vi "Reset To Temporary Passwordvi.vi"(0 "User Configuration Manager in":refnum<class "User Configuration Manager.lvclass">, 5 "Username":string, 11 "error in (no error)":errorcluster) -> (4 "User Configuration Manager out":refnum<class "User Configuration Manager.lvclass">, 6 "User Found":bool, 8 "Temporary Password":string, 15 "error out":errorcluster)   [LabVIEW 2020, in "User Configuration Manager.lvlib" / "User Configuration Manager.lvclass"]
doc: "Resets the password of the user specified by user name to a temporary password."
uses:
  <vilib>/gpm_packages/@cs/user-manager/Source/User Configuration Manager/User Configuration Manager.lvclass
  <vilib>/gpm_packages/@cs/user-manager/Source/User Configuration Manager/User Configuration Manager.lvclass/User Configuration Manager.ctl
  1ef86e87-005e-4bc9-afcc-fd6cee3e8d09.vi
  <vilib>/gpm_packages/@cs/user-manager/Source/User Configuration Manager/Accessors/Read Linked List Ref .vi
  <vilib>/gpm_packages/@cs/user-manager/Source/User Configuration Manager/Read Encryption Type.vi
  <vilib>/gpm_packages/@cs/linked-list/Source/Linked List/ILinkedList/ILinked List.lvclass
  <vilib>/gpm_packages/@cs/user-manager/Source/iEncryption/iEncryption.lvclass
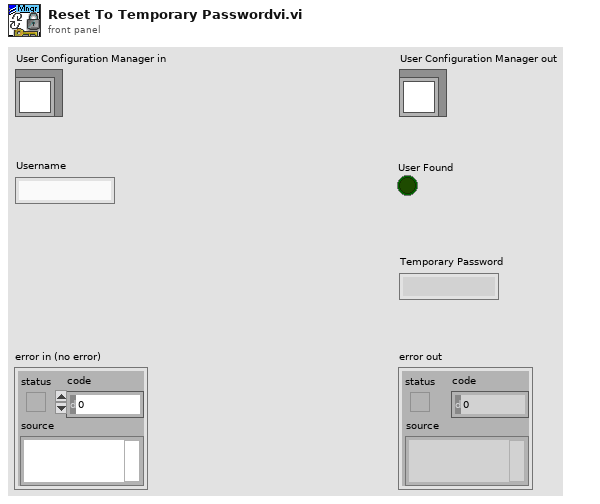
[diagram p1: front panel]
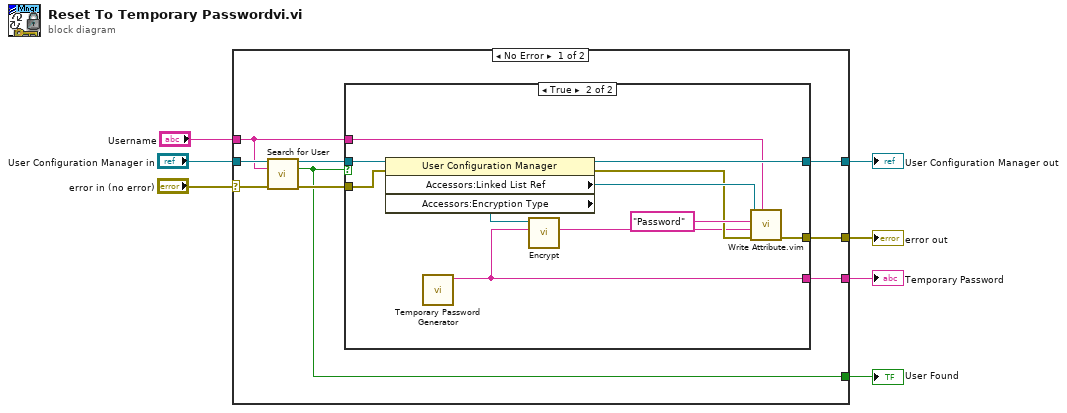
[diagram p0: block diagram]
diagram:
  n1 = case shown="No Error" "error in (no error)" {
    selector: "error in (no error)" -> [w10 w30]
    tunnel: "User Configuration Manager in" -> [w13 w31]
    tunnel: "Username" -> [w9 _]
    tunnel: [w16 w31] -> w4
    tunnel: [w15 w30] -> w3
    tunnel: [w14 _] -> w2
    tunnel: [w8 _] -> w1
    frame No Error {
      n2 = call-dynamic "Search for User.vi"("User Configuration Manager in"=w13, "Username"=w9, "error in (no error)"=w10) -> ("User Configuration Manager out"=w12:refnum<class "User Configuration Manager.lvclass">, "Found"=w8:bool, "error out"=w11:errorcluster)  [unwired: 10 in]
      n3 = case shown="True" w8 {
        tunnel: [w18 w29] -> w16
        tunnel: [w17 w27] -> w15
        tunnel: [_ w19] -> w14
        tunnel: w12 -> [w18 w25]
        tunnel: w11 -> [w17 w24]
        tunnel: w9 -> [_ w23]
        frame False {
        }
        frame True {
          n4 = property class="User Configuration Manager"(reference=w25, error in=w24) -> (reference out=w29:refnum<class "User Configuration Manager.lvclass">, error out=w22:errorcluster, "Accessors:Linked List Ref "=w26:refnum<data-value>, "Accessors:Encryption Type"=w21:refnum<class "iEncryption.lvclass">)
          n5 = call <vilib>:"Temporary Password Generator.vi"() -> ("Temporary Password"=w19:string)  [unwired: 11 in]
          n6 = call-dynamic "Encrypt.vi"("String"=w19, "iEncryption in"=w21) -> ("Encrypted String"=w20:string)  [unwired: 9 in]
          n7 = call "Write Attribute.vim"("Linked List ID"=w23, "error in (no error)"=w22, "Attribute"=w20, "Attribute Name"="Password", "Linked List Ref"=w26) -> ("error out"=w27:errorcluster)  [unwired: 3 in, 3 out]
        }
      }
    }
    frame Error {
    }
  }
  "error out" <- w3
  "User Configuration Manager out" <- w4
  "Temporary Password" <- w2
  "User Found" <- w1
